vi "ActKeyboardSearch.vi"(8 "Error":errorcluster, 10 "ChatId":i32, 11 "ActKeyboards in":cluster{"ChatId":i32, "Cmd":string}[](array[cluster])) -> (0 "Error":errorcluster, 1 "Offset":i32, 2 "Cmd":string, 3 "ActKeyboards out":cluster{"ChatId":i32, "Cmd":string}[](array[cluster]))   [LabVIEW 2015]
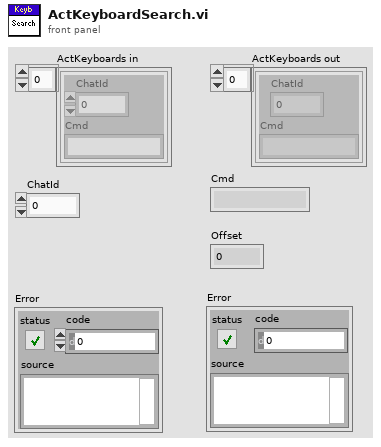
[diagram p1: front panel]
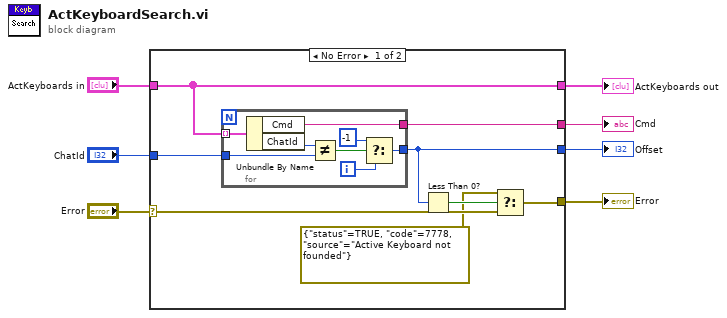
[diagram p0: block diagram]
diagram:
  n1 = case shown="No Error" "Error" {
    selector: "Error" -> [w11 w25]
    tunnel: [w8 w24] -> w1
    tunnel: "ActKeyboards in" -> [w8 w24]
    tunnel: [w13 _] -> w7
    tunnel: [w15 _] -> w6
    tunnel: "ChatId" -> [w14 _]
    tunnel: [w9 w25] -> w3
    frame No Error {
      n2 = for {
        tunnel: w8 -> [w23] mode=indexing
        tunnel: [w22] -> w15
        tunnel: w14 -> [w21]
        tunnel: [w16] -> w13
        i -> [w18]
        n3 = Unbundle By Name(w23) -> ("Cmd"=w22:string, "ChatId"=w19:i32)
        n4 = Not Equal?(x=w19, y=w21) -> (x != y?=w20:bool)
        n5 = Select(t=-1, s=w20, f=w18) -> (s? t:f=w16:i32)
      }
      n6 = Less Than 0?(x=w13) -> (x < 0?=w12:bool)
      n7 = Select(t=errorcluster {"status"=TRUE, "code"=7778, "source"="Active Keyboard not founded"}, s=w12, f=w11) -> (s? t:f=w9:errorcluster)
    }
    frame Error {
    }
  }
  "Cmd" <- w6
  "Offset" <- w7
  "Error" <- w3
  "ActKeyboards out" <- w1
